vi "Template Path.vi"() -> (3 "path":path)   [LabVIEW 2016]
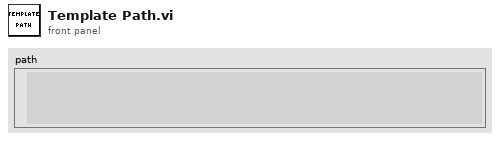
[diagram p1: front panel]
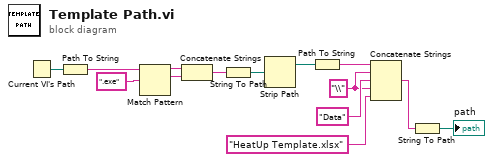
[diagram p0: block diagram]
diagram:
  w5 = "\\" ("string")
  n1 = Current VI's Path() -> (path=w1:path)
  n2 = Path To String(path=w1) -> (string=w14:string)
  n3 = Match Pattern(string=w14, regular expression=".exe") -> (before substring=w12:string, match substring=w11:string)  [unwired: 1 in, 2 out]
  n4 = Concatenate Strings(w12, w11) -> (w10:string)
  n5 = String To Path(string=w10) -> (path=w9:path)
  n6 = Strip Path(path=w9) -> (stripped path=w8:path)  [unwired: 1 out]
  n7 = Path To String(path=w8) -> (string=w7:string)
  n8 = Concatenate Strings(w7, w5, "Data" ("string"), w5, "HeatUp Template.xlsx" ("string")) -> (w3:string)
  n9 = String To Path(string=w3) -> (path=→"path":path)
